vi "ViChoice_test.vi"() -> ()   [LabVIEW 2015]
uses:
  GlobalPath.vi
  GlobalVi.vi
  GlobalData.vi
panel:
  out "Finalization":bool
  out "element":string
  out "NewPanel 3":bool
  in  "Restart from scratch?":bool
  out "Lines":string[](array[string])
  out "PinInsertGlue":bool
  out "QAQCvacoff":bool
  out "StiffRemoval":bool
  out "QAQCvacon":bool
  out "DrunRunFull":bool
  out "AllCoolBar":bool
  out "AddHoneycomb":bool
  out "AddFrame":bool
  out "PCBalignStiff":bool
  out "PCBposStiff":bool
  out "PCBalignTab":bool
  out "NewPanel":bool
  in  "Construction Finalization":bool
  in  "Panel QA/QC vacuum off":bool
  in  "Gluing of alignment pin/insert":bool
  in  "Panel QA/QC vacuum on":bool
  in  "Stiffback removal":bool
  in  "Add Cooling Bars":bool
  in  "Add Honeycomb":bool
  in  "Add Frames":bool
  in  "Dry Run (full)":bool
  in  "PCB Alignment on stiffback":bool
  in  "PCB Positioning on stiffback":bool
  in  "PCB Alignment on table":bool
  in  "New Panel":bool
  in  "current vi path":path
  out "Opening program":string
  in  "PCB gluing on table":bool
  in  "Internal structure positioning":bool
  in  "Stiffback gluing":bool
  in  "PCB Positioning on table":bool
  in  "Panel Closure":bool
  out "closePanel":bool
  out "PCBposTab":bool
  out "stbackPCBglue":bool
  out "tablePCBglue":bool
  out "innerStructure":bool
  # "Status"
  # "Control"
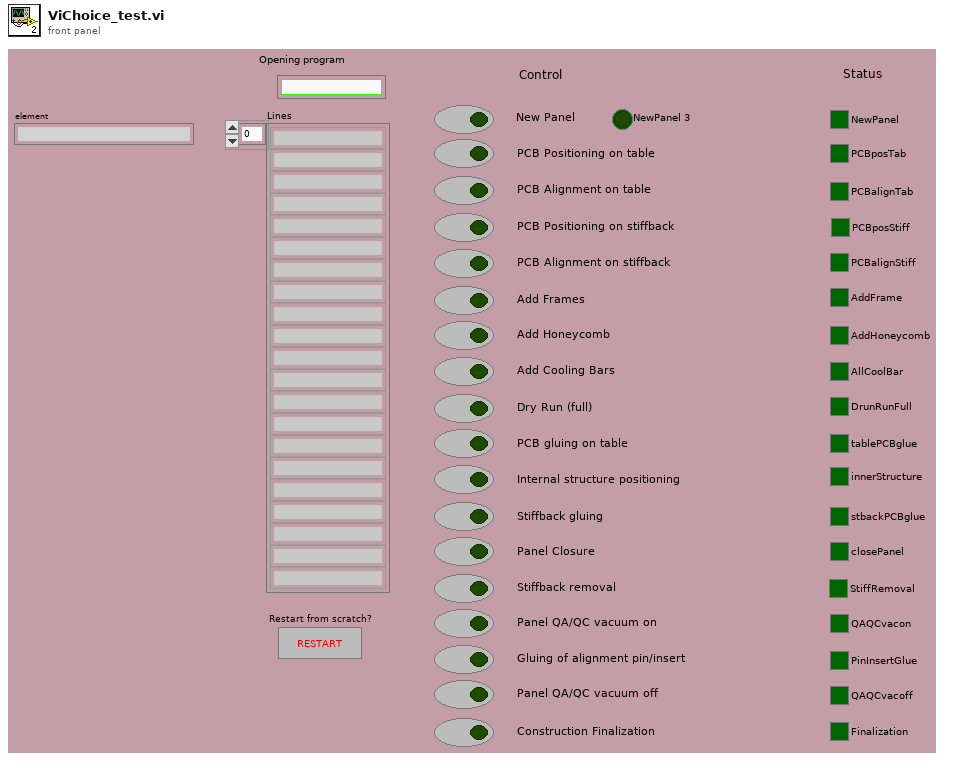
[diagram p1: front panel]
types:
  T1 = enum16{"open", "replace", "create", "open or create", "replace or create", "replace or create with confirmation"}
  T2 = cluster{"top":i32, "left":i32, "bottom":i32, "right":i32}
  T3 = enum32{"Bad", "Idle", "Run top level", "Running"}
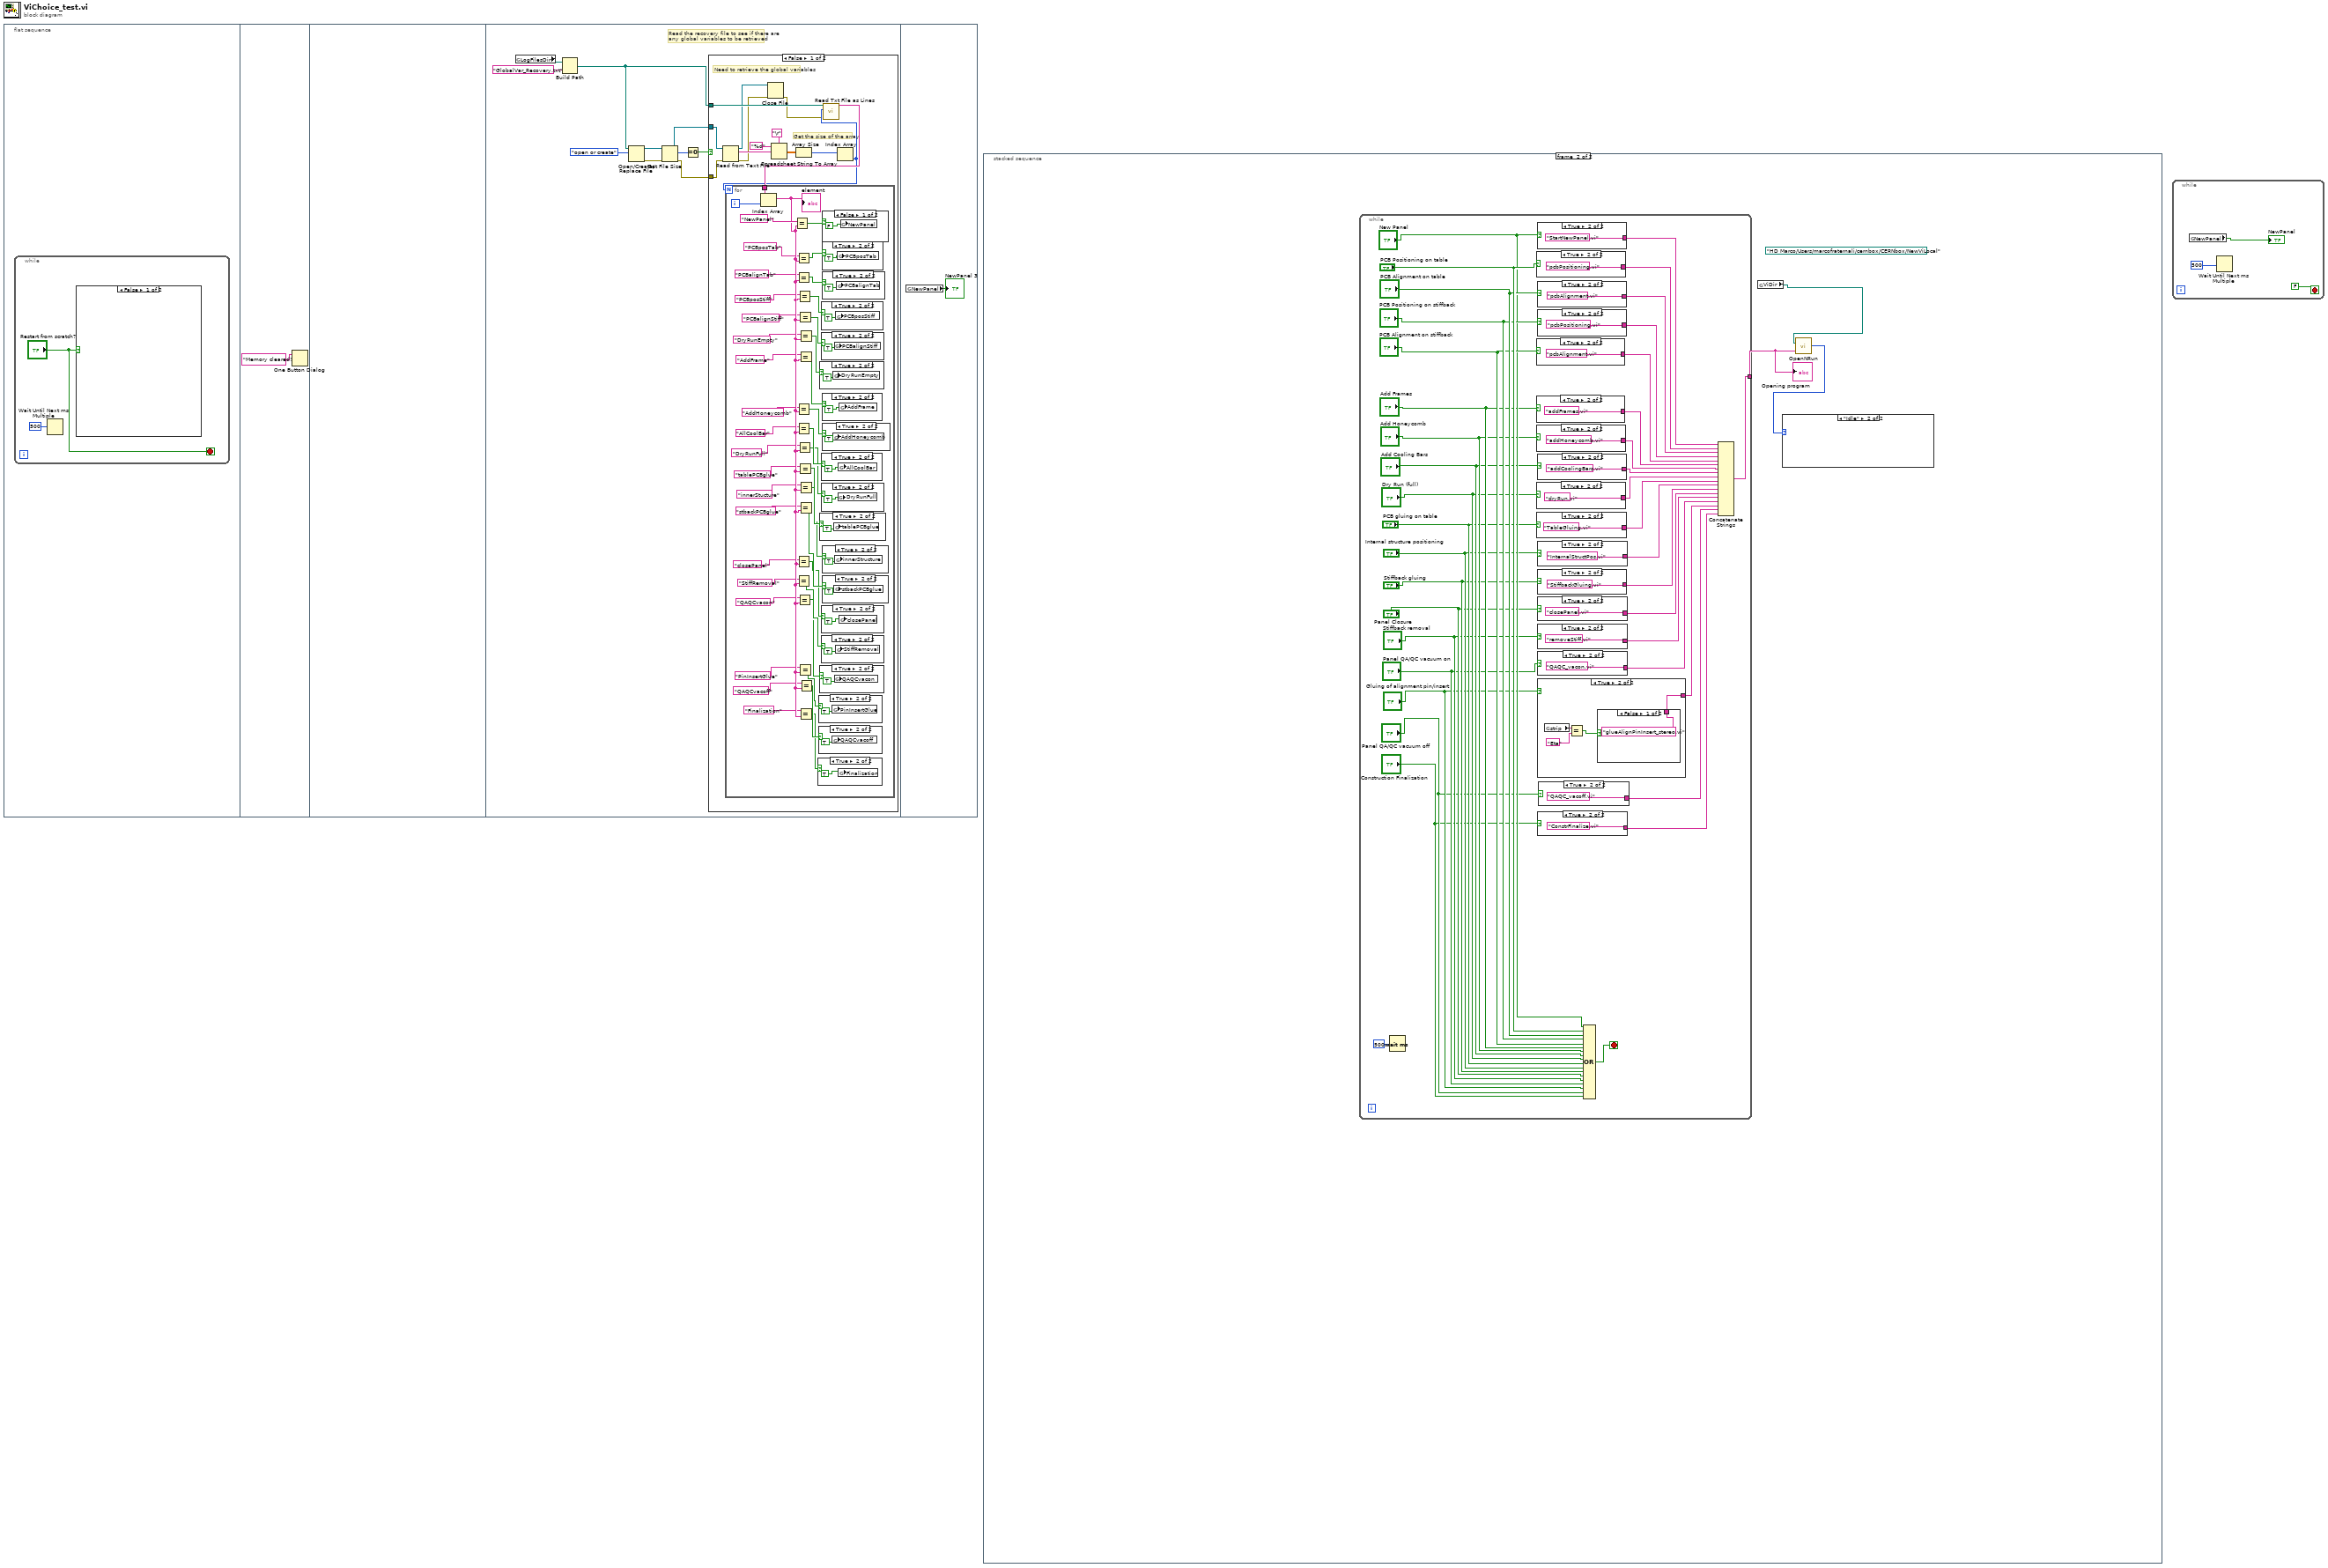
[diagram p0: block diagram]
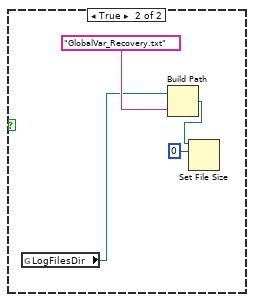
[diagram p2: hidden frame]
diagram:
  n1 = flat-sequence {
    frame #0 {
      n2 = while {
        stop <- "Restart from scratch?" stop-if-true
        n3 = Wait Until Next ms Multiple(millisecond multiple=u32 500) -> ()  [unwired: 1 out]
        n4 = case shown="False" "Restart from scratch?" {
          frame False {
          }
          frame True {
            n5 = global read "GlobalPath.vi" "LogFilesDir"() -> (w5:path)
            n6 = Build Path(base path=w5, name or relative path="GlobalVar_Recovery.txt") -> (appended path=w4:path)
            n7 = Set File Size(6:0, 7:w4) -> ()  [unwired: 1 in, 2 out]
          }
        }
      }
    }
    frame #1 {
      n8 = One Button Dialog(message="Memory cleared!") -> ()  [unwired: 1 in, 1 out]
    }
    frame #2 {
    }
    frame #3 {
      # "Read the recovery file to see if there are\nany global variables to be retrieved"
      n9 = global read "GlobalPath.vi" "LogFilesDir"() -> (w8:path)
      n10 = Build Path(base path=w8, name or relative path="GlobalVar_Recovery.txt") -> (appended path=w9:path)
      n11 = Open/Create/Replace File(file path (use dialog)=w9, operation (0:open)=T1."open or create") -> (refnum out=w16:refnum<file>, error out=w14:errorcluster)  [unwired: 4 in, 1 out]
      n12 = Get File Size(file=w16, error in=w14) -> (refnum out=w12:refnum<file>, size (in bytes)=w15:i64, 0:w11:errorcluster)
      n13 = Equal To 0?(x=w15) -> (x = 0?=w13:bool)
      n14 = case shown="False" w13 {
        tunnel: w12 -> [w25 _]
        tunnel: w11 -> [w27 _]
        tunnel: w9 -> [w24 _]
        frame False {
          # "Get the size of the array"
          # "Need to retrieve the global variables"
          n15 = Read from Text File(file (use dialog)=w25, error in=w27) -> (refnum out=w20:refnum<file>, text=w28:string, error out=w19:errorcluster)  [unwired: 3 out]
          n16 = Close File(refnum=w20, error in=w19) -> (error out=w18:errorcluster)  [unwired: 1 out]
          n17 = Spreadsheet String To Array(delimiter (Tab)="\r", format string="%d", spreadsheet string=w28) -> (array=w26:dbl[][])  [unwired: 1 out]
          n18 = Array Size(array=w26) -> (size(s)=w23:i32[])
          n19 = Index Array(array=w23) -> (element=w21:i32)  [unwired: 1 in]
          n20 = call "Read Txt File as Lines.vi"("error in"=w18, "Lines to Read"=w21, "file path (use dialog)"=w24) -> ("Lines"=w22:string[])  [unwired: 7 in, 1 out]
          n21 = for {
            N: w21 -> [_]
            tunnel: w22 -> [w71]
            i -> [w31]
            n22 = Index Array(array=w71, index=w31) -> (element=w50:string)
            "element" <- w50
            n23 = Equal?(x="NewPanel", y=w50) -> (x = y?=w70:bool)
            n24 = Equal?(x="PCBposTab", y=w50) -> (x = y?=w69:bool)
            n25 = Equal?(x="PCBalignTab", y=w50) -> (x = y?=w68:bool)
            n26 = Equal?(x="AddHoneycomb", y=w50) -> (x = y?=w63:bool)
            n27 = Equal?(x="AllCoolBar", y=w50) -> (x = y?=w62:bool)
            n28 = Equal?(x="closePanel", y=w50) -> (x = y?=w57:bool)
            n29 = Equal?(x="StiffRemoval", y=w50) -> (x = y?=w56:bool)
            n30 = Equal?(x="PCBposStiff", y=w50) -> (x = y?=w67:bool)
            n31 = Equal?(x="DryRunFull", y=w50) -> (x = y?=w61:bool)
            n32 = Equal?(x="QAQCvacon", y=w50) -> (x = y?=w55:bool)
            n33 = Equal?(x="PCBalignStiff", y=w50) -> (x = y?=w66:bool)
            n34 = Equal?(x="tablePCBglue", y=w50) -> (x = y?=w60:bool)
            n35 = Equal?(x="PinInsertGlue", y=w50) -> (x = y?=w54:bool)
            n36 = Equal?(x="DryRunEmpty", y=w50) -> (x = y?=w65:bool)
            n37 = Equal?(x="AddFrame", y=w50) -> (x = y?=w64:bool)
            n38 = Equal?(x="innerStucture", y=w50) -> (x = y?=w59:bool)
            n39 = Equal?(x="stbackPCBglue", y=w50) -> (x = y?=w58:bool)
            n40 = Equal?(x="Finalization", y=w50) -> (x = y?=w52:bool)
            n41 = Equal?(x="QAQCvacoff", y=w50) -> (x = y?=w53:bool)
            n42 = case shown="True" w52 {
              frame False {
              }
              frame True {
                n43 = global write "GlobalVi.vi" "Finalization"(TRUE) -> ()
              }
            }
            n44 = case shown="True" w54 {
              frame False {
              }
              frame True {
                n45 = global write "GlobalVi.vi" "PinInsertGlue"(TRUE) -> ()
              }
            }
            n46 = case shown="True" w53 {
              frame False {
              }
              frame True {
                n47 = global write "GlobalVi.vi" "QAQCvacoff"(TRUE) -> ()
              }
            }
            n48 = case shown="True" w65 {
              frame False {
              }
              frame True {
                n49 = global write "GlobalVi.vi" "DryRunEmpty"(TRUE) -> ()
              }
            }
            n50 = case shown="True" w60 {
              frame False {
              }
              frame True {
                n51 = global write "GlobalVi.vi" "tablePCBglue"(TRUE) -> ()
              }
            }
            n52 = case shown="True" w55 {
              frame False {
              }
              frame True {
                n53 = global write "GlobalVi.vi" "QAQCvacon"(TRUE) -> ()
              }
            }
            n54 = case shown="True" w66 {
              frame False {
              }
              frame True {
                n55 = global write "GlobalVi.vi" "PCBalignStiff"(TRUE) -> ()
              }
            }
            n56 = case shown="True" w61 {
              frame False {
              }
              frame True {
                n57 = global write "GlobalVi.vi" "DryRunFull"(TRUE) -> ()
              }
            }
            n58 = case shown="True" w56 {
              frame False {
              }
              frame True {
                n59 = global write "GlobalVi.vi" "StiffRemoval"(TRUE) -> ()
              }
            }
            n60 = case shown="True" w67 {
              frame False {
              }
              frame True {
                n61 = global write "GlobalVi.vi" "PCBposStiff"(TRUE) -> ()
              }
            }
            n62 = case shown="True" w62 {
              frame False {
              }
              frame True {
                n63 = global write "GlobalVi.vi" "AllCoolBar"(TRUE) -> ()
              }
            }
            n64 = case shown="True" w57 {
              frame False {
              }
              frame True {
                n65 = global write "GlobalVi.vi" "closePanel"(TRUE) -> ()
              }
            }
            n66 = case shown="False" w70 {
              frame False {
                n67 = global write "GlobalVi.vi" "NewPanel"(FALSE) -> ()
              }
              frame True {
                n68 = global write "GlobalVi.vi" "NewPanel"(TRUE) -> ()
              }
            }
            n69 = case shown="True" w69 {
              frame False {
              }
              frame True {
                n70 = global write "GlobalVi.vi" "PCBposTab"(TRUE) -> ()
              }
            }
            n71 = case shown="True" w68 {
              frame False {
              }
              frame True {
                n72 = global write "GlobalVi.vi" "PCBalignTab"(TRUE) -> ()
              }
            }
            n73 = case shown="True" w64 {
              frame False {
              }
              frame True {
                n74 = global write "GlobalVi.vi" "AddFrame"(TRUE) -> ()
              }
            }
            n75 = case shown="True" w63 {
              frame False {
              }
              frame True {
                n76 = global write "GlobalVi.vi" "AddHoneycomb"(TRUE) -> ()
              }
            }
            n77 = case shown="True" w59 {
              frame False {
              }
              frame True {
                n78 = global write "GlobalVi.vi" "innerStructure"(TRUE) -> ()
              }
            }
            n79 = case shown="True" w58 {
              frame False {
              }
              frame True {
                n80 = global write "GlobalVi.vi" "stbackPCBglue"(TRUE) -> ()
              }
            }
          }
        }
        frame True {
          # "File is empty so nothing to retrieve"
        }
      }
    }
    frame #4 {
      n81 = global read "GlobalVi.vi" "NewPanel"() -> (→"NewPanel 3":bool)
    }
  }
  n82 = stacked-sequence {
    frame #0 {
      n83 = flat-sequence {
        frame #0 {
          n84 = call <vilib>:"Get System Directory.vi"("system directory type"=0) -> ("system directory"=w95:path)  [unwired: 10 in]
          n85 = Build Path(base path=w95, name or relative path="Micromegas/interface") -> (appended path=w94:path)
          n86 = Build Path(base path=w95, name or relative path="Micromegas/M05Data/logfiles") -> (appended path=w96:path)
          n87 = global write "GlobalPath.vi" "ViDir"(w94) -> ()
          n88 = global write "GlobalPath.vi" "LogFilesDir"(w96) -> ()
        }
        frame #1 {
          (unwired) path "/HD Marco/Users/marcofraternali/Desktop" ("path")
          # "Read the recovery file to see if there are\nany global variables to be retrieved"
          n89 = global read "GlobalPath.vi" "LogFilesDir"() -> (w99:path)
          n90 = Build Path(base path=w99, name or relative path="GlobalVar_Recovery.txt") -> (appended path=w100:path)
          n91 = Open/Create/Replace File(file path (use dialog)=w100, operation (0:open)=T1."open or create") -> (refnum out=w107:refnum<file>, error out=w105:errorcluster)  [unwired: 4 in, 1 out]
          n92 = Get File Size(file=w107, error in=w105) -> (refnum out=w103:refnum<file>, size (in bytes)=w106:i64, 0:w102:errorcluster)
          n93 = Equal To 0?(x=w106) -> (x = 0?=w104:bool)
          n94 = case shown="False" w104 {
            tunnel: w103 -> [w116 _]
            tunnel: w102 -> [w118 _]
            tunnel: w100 -> [w115 _]
            frame False {
              # "Get the size of the array"
              # "Need to retrieve the global variables"
              n95 = Read from Text File(file (use dialog)=w116, error in=w118) -> (refnum out=w111:refnum<file>, text=w119:string, error out=w110:errorcluster)  [unwired: 3 out]
              n96 = Close File(refnum=w111, error in=w110) -> (error out=w109:errorcluster)  [unwired: 1 out]
              n97 = Spreadsheet String To Array(delimiter (Tab)="\r", format string="%d", spreadsheet string=w119) -> (array=w117:dbl[][])  [unwired: 1 out]
              n98 = Array Size(array=w117) -> (size(s)=w114:i32[])
              n99 = Index Array(array=w114) -> (element=w112:i32)  [unwired: 1 in]
              n100 = call "Read Txt File as Lines.vi"("error in"=w109, "Lines to Read"=w112, "file path (use dialog)"=w115) -> ("Lines"=w113:string[])  [unwired: 7 in, 1 out]
              "Lines" <- w113
              n101 = for {
                N: w112 -> [_]
                tunnel: w113 -> [w162]
                i -> [w122]
                n102 = Index Array(array=w162, index=w122) -> (element=w141:string)
                n103 = Equal?(x="NewPanel", y=w141) -> (x = y?=w161:bool)
                n104 = Equal?(x="PCBposTab", y=w141) -> (x = y?=w160:bool)
                n105 = Equal?(x="PCBalignTab", y=w141) -> (x = y?=w159:bool)
                n106 = Equal?(x="AddHoneycomb", y=w141) -> (x = y?=w154:bool)
                n107 = Equal?(x="AllCoolBar", y=w141) -> (x = y?=w153:bool)
                n108 = Equal?(x="closePanel", y=w141) -> (x = y?=w148:bool)
                n109 = Equal?(x="StiffRemoval", y=w141) -> (x = y?=w147:bool)
                n110 = Equal?(x="PCBposStiff", y=w141) -> (x = y?=w158:bool)
                n111 = Equal?(x="DryRunFull", y=w141) -> (x = y?=w152:bool)
                n112 = Equal?(x="QAQCvacon", y=w141) -> (x = y?=w146:bool)
                n113 = Equal?(x="PCBalignStiff", y=w141) -> (x = y?=w157:bool)
                n114 = Equal?(x="tablePCBglue", y=w141) -> (x = y?=w151:bool)
                n115 = Equal?(x="PinInsertGlue", y=w141) -> (x = y?=w145:bool)
                n116 = Equal?(x="DryRunEmpty", y=w141) -> (x = y?=w156:bool)
                n117 = Equal?(x="AddFrame", y=w141) -> (x = y?=w155:bool)
                n118 = Equal?(x="innerStucture", y=w141) -> (x = y?=w150:bool)
                n119 = Equal?(x="stbackPCBglue", y=w141) -> (x = y?=w149:bool)
                n120 = Equal?(x="Finalization", y=w141) -> (x = y?=w143:bool)
                n121 = Equal?(x="QAQCvacoff", y=w141) -> (x = y?=w144:bool)
                n122 = case shown="True" w143 {
                  frame False {
                  }
                  frame True {
                    n123 = global write "GlobalVi.vi" "Finalization"(TRUE) -> ()
                  }
                }
                n124 = case shown="True" w145 {
                  frame False {
                  }
                  frame True {
                    n125 = global write "GlobalVi.vi" "PinInsertGlue"(TRUE) -> ()
                  }
                }
                n126 = case shown="True" w144 {
                  frame False {
                  }
                  frame True {
                    n127 = global write "GlobalVi.vi" "QAQCvacoff"(TRUE) -> ()
                  }
                }
                n128 = case shown="True" w156 {
                  frame False {
                  }
                  frame True {
                    n129 = global write "GlobalVi.vi" "DryRunEmpty"(TRUE) -> ()
                  }
                }
                n130 = case shown="True" w151 {
                  frame False {
                  }
                  frame True {
                    n131 = global write "GlobalVi.vi" "tablePCBglue"(TRUE) -> ()
                  }
                }
                n132 = case shown="True" w146 {
                  frame False {
                  }
                  frame True {
                    n133 = global write "GlobalVi.vi" "QAQCvacon"(TRUE) -> ()
                  }
                }
                n134 = case shown="True" w157 {
                  frame False {
                  }
                  frame True {
                    n135 = global write "GlobalVi.vi" "PCBalignStiff"(TRUE) -> ()
                  }
                }
                n136 = case shown="True" w152 {
                  frame False {
                  }
                  frame True {
                    n137 = global write "GlobalVi.vi" "DryRunFull"(TRUE) -> ()
                  }
                }
                n138 = case shown="True" w147 {
                  frame False {
                  }
                  frame True {
                    n139 = global write "GlobalVi.vi" "StiffRemoval"(TRUE) -> ()
                  }
                }
                n140 = case shown="True" w158 {
                  frame False {
                  }
                  frame True {
                    n141 = global write "GlobalVi.vi" "PCBposStiff"(TRUE) -> ()
                  }
                }
                n142 = case shown="True" w153 {
                  frame False {
                  }
                  frame True {
                    n143 = global write "GlobalVi.vi" "AllCoolBar"(TRUE) -> ()
                  }
                }
                n144 = case shown="True" w148 {
                  frame False {
                  }
                  frame True {
                    n145 = global write "GlobalVi.vi" "closePanel"(TRUE) -> ()
                  }
                }
                n146 = case shown="False" w161 {
                  frame False {
                    n147 = global write "GlobalVi.vi" "NewPanel"(FALSE) -> ()
                  }
                  frame True {
                    n148 = global write "GlobalVi.vi" "NewPanel"(TRUE) -> ()
                  }
                }
                n149 = case shown="True" w160 {
                  frame False {
                  }
                  frame True {
                    n150 = global write "GlobalVi.vi" "PCBposTab"(TRUE) -> ()
                  }
                }
                n151 = case shown="True" w159 {
                  frame False {
                  }
                  frame True {
                    n152 = global write "GlobalVi.vi" "PCBalignTab"(TRUE) -> ()
                  }
                }
                n153 = case shown="True" w155 {
                  frame False {
                  }
                  frame True {
                    n154 = global write "GlobalVi.vi" "AddFrame"(TRUE) -> ()
                  }
                }
                n155 = case shown="True" w154 {
                  frame False {
                  }
                  frame True {
                    n156 = global write "GlobalVi.vi" "AddHoneycomb"(TRUE) -> ()
                  }
                }
                n157 = case shown="True" w150 {
                  frame False {
                  }
                  frame True {
                    n158 = global write "GlobalVi.vi" "innerStructure"(TRUE) -> ()
                  }
                }
                n159 = case shown="True" w149 {
                  frame False {
                  }
                  frame True {
                    n160 = global write "GlobalVi.vi" "stbackPCBglue"(TRUE) -> ()
                  }
                }
              }
            }
            frame True {
              # "File is empty so nothing to retrieve"
            }
          }
        }
        frame #2 {
          # "In the beginning of the program we check which of all the steps are done (through global variables)"
          n161 = Current VI's Path() -> (path=w204:path)
          n162 = Current VI's Path() -> (path=w206:path)
          n163 = global read "GlobalVi.vi" "dimbig"() -> (w202:T2)
          n164 = Strip Path(path=w204) -> (name=w203:string)  [unwired: 1 out]
          n165 = Strip Path(path=w206) -> (name=w195:string)  [unwired: 1 out]
          n166 = Wait (ms)(milliseconds to wait=u32 500) -> ()  [unwired: 1 out]
          n167 = call <vilib>:"Resize Panel.vi"("panel location and size"=w202, "VI name"=w203) -> ()  [unwired: 9 in, 1 out]
          n168 = local write "Opening program"("") -> ()
          n169 = global write "GlobalData.vi" "programma"(w195) -> ()
          n170 = global read "GlobalVi.vi" "QAQCvacoff"() -> (→"QAQCvacoff":bool)
          n171 = global read "GlobalVi.vi" "AddHoneycomb"() -> (→"AddHoneycomb":bool)
          n172 = global read "GlobalVi.vi" "DryRunFull"() -> (→"DrunRunFull":bool)
          n173 = global read "GlobalVi.vi" "tablePCBglue"() -> (→"tablePCBglue":bool)
          n174 = global read "GlobalVi.vi" "stbackPCBglue"() -> (→"stbackPCBglue":bool)
          n175 = global read "GlobalVi.vi" "closePanel"() -> (→"closePanel":bool)
          n176 = global read "GlobalVi.vi" "QAQCvacon"() -> (→"QAQCvacon":bool)
          n177 = global read "GlobalVi.vi" "innerStructure"() -> (→"innerStructure":bool)
          n178 = global read "GlobalVi.vi" "PinInsertGlue"() -> (→"PinInsertGlue":bool)
          n179 = global read "GlobalVi.vi" "PCBalignStiff"() -> (→"PCBalignStiff":bool)
          n180 = global read "GlobalVi.vi" "AllCoolBar"() -> (→"AllCoolBar":bool)
          n181 = global read "GlobalVi.vi" "StiffRemoval"() -> (→"StiffRemoval":bool)
          n182 = global read "GlobalVi.vi" "PCBalignTab"() -> (→"PCBalignTab":bool)
          n183 = global read "GlobalVi.vi" "PCBposStiff"() -> (→"PCBposStiff":bool)
          n184 = global read "GlobalVi.vi" "AddFrame"() -> (→"AddFrame":bool)
          n185 = global read "GlobalVi.vi" "Finalization"() -> (→"Finalization":bool)
          n186 = global read "GlobalVi.vi" "PCBposTab"() -> (→"PCBposTab":bool)
        }
      }
    }
    frame #1 {
      (unwired) path "/HD Marco/Users/marcofraternali/cernbox/CERNbox/NewViLocal" ("path")
      n187 = while {
        tunnel: [w251] -> w209
        stop <- w252 stop-if-true
        n188 = Wait (ms)(milliseconds to wait=u32 500) -> ()  [unwired: 1 out]
        n189 = case shown="True" "PCB Alignment on stiffback" {
          tunnel: ["" "pcbAlignment.vi"] -> w246
          frame False {
          }
          frame True {
          }
        }
        n190 = case shown="True" "Add Frames" {
          tunnel: ["" "addFrames.vi"] -> w240
          frame False {
          }
          frame True {
          }
        }
        n191 = case shown="True" "PCB Positioning on table" {
          tunnel: ["" "pcbPositioning.vi"] -> w250
          frame False {
          }
          frame True {
          }
        }
        n192 = case shown="True" "Add Honeycomb" {
          tunnel: ["" "addHoneycomb.vi"] -> w239
          frame False {
          }
          frame True {
          }
        }
        n193 = case shown="True" "Dry Run (full)" {
          tunnel: ["" "dryRun.vi"] -> w237
          frame False {
          }
          frame True {
          }
        }
        n194 = case shown="True" "PCB gluing on table" {
          tunnel: ["" "TableGluing.vi"] -> w236
          frame False {
          }
          frame True {
          }
        }
        n195 = case shown="True" "PCB Alignment on table" {
          tunnel: ["" "pcbAlignment.vi"] -> w248
          frame False {
          }
          frame True {
          }
        }
        n196 = case shown="True" "PCB Positioning on stiffback" {
          tunnel: ["" "pcbPositioning.vi"] -> w247
          frame False {
          }
          frame True {
          }
        }
        n197 = case shown="True" "Add Cooling Bars" {
          tunnel: ["" "addCoolingBars.vi"] -> w238
          frame False {
          }
          frame True {
          }
        }
        n198 = case shown="True" "Internal structure positioning" {
          tunnel: ["" "InternalStructPos.vi"] -> w235
          frame False {
          }
          frame True {
          }
        }
        n199 = case shown="True" "Stiffback gluing" {
          tunnel: ["" "StiffbackGluing.vi"] -> w234
          frame False {
          }
          frame True {
          }
        }
        n200 = case shown="True" "Panel Closure" {
          tunnel: ["" "closePanel.vi"] -> w233
          frame False {
          }
          frame True {
          }
        }
        n201 = case shown="True" "Stiffback removal" {
          tunnel: ["" "removeStiff.vi"] -> w232
          frame False {
          }
          frame True {
          }
        }
        n202 = case shown="True" "New Panel" {
          tunnel: ["" "StartNewPanel.vi"] -> w249
          frame False {
          }
          frame True {
          }
        }
        n203 = case shown="True" "Panel QA/QC vacuum on" {
          tunnel: ["" "QAQC_vacon.vi"] -> w231
          frame False {
          }
          frame True {
          }
        }
        n204 = case shown="True" "Gluing of alignment pin/insert" {
          tunnel: ["" w262] -> w230
          frame False {
          }
          frame True {
            n205 = global read "GlobalData.vi" "strip"() -> (w261:string)
            n206 = Equal?(x=w261, y="Eta") -> (x = y?=w259:bool)
            n207 = case shown="False" w259 {
              tunnel: ["glueAlignPinInsert_stereo.vi" "glueAlignPinInsert.vi"] -> w262
              frame False {
              }
              frame True {
              }
            }
          }
        }
        n208 = case shown="True" "Construction Finalization" {
          tunnel: ["" "ConstrFinalize.vi"] -> w228
          frame False {
          }
          frame True {
          }
        }
        n209 = case shown="True" "Panel QA/QC vacuum off" {
          tunnel: ["" "QAQC_vacoff.vi"] -> w229
          frame False {
          }
          frame True {
          }
        }
        n210 = Compound Arithmetic op=OR("New Panel", "PCB Positioning on table", "PCB Alignment on table", "PCB Positioning on stiffback", "PCB Alignment on stiffback", "Add Frames", "Add Honeycomb", "Add Cooling Bars", "Dry Run (full)", "PCB gluing on table", "Internal structure positioning", "Stiffback gluing", "Panel Closure", "Stiffback removal", "Panel QA/QC vacuum on", "Gluing of alignment pin/insert", "Panel QA/QC vacuum off", "Construction Finalization") -> (w252:bool)
        n211 = Concatenate Strings(w249, w250, w248, w247, w246, w240, w239, w238, w237, w236, w235, w234, w233, w232, w231, w230, w229, w228) -> (w251:string)
      }
      "Opening program" <- w209
      n212 = global read "GlobalPath.vi" "ViDir"() -> (w207:path)
      n213 = call "OpenNRun.vi"("VI name"=w209, "ViDirPath"=w207) -> ("Execution:State"=w208:T3)
      n214 = case shown="\"Idle\"" w208 {
        frame "Bad", Default {
          n215 = Open VI Reference(vi path="current vi path") -> (vi reference=w214:refnum<vi>, error out=w213:errorcluster)  [unwired: 5 in]
          n216 = global read "GlobalPath.vi" "ViDir"() -> (w211:path)
          n217 = property class="VI"(reference=w214, error in=w213) -> ("Name"=w210:string)  [unwired: 2 out]
          n218 = call "OpenNRun.vi"("VI name"=w210, "ViDirPath"=w211) -> ()  [unwired: 1 out]
        }
        frame "Idle" {
        }
      }
    }
  }
  n219 = while {
    stop <- FALSE stop-if-true
    n220 = global read "GlobalVi.vi" "NewPanel"() -> (→"NewPanel":bool)
    n221 = Wait Until Next ms Multiple(millisecond multiple=500) -> ()  [unwired: 1 out]
  }
